vi "Linear Ramp (DBL).vi"(6 "Options":T1, 9 "Delta":dbl, 10 "Max":dbl, 11 "Min":dbl) -> (1 "# Elements":i32, 3 "Ramp":dbl[](array[numeric]))   [LabVIEW 2021, in "Arrays.lvlib"]
doc: "Creates a linear ramp with steps provided by \"Delta\".\nDepending on the chosen Options:\n\n- Include Min/Exclude Max (Default)\n- Exclude Min/Include Max\n- Include Both\n- Exclude Both\n\nthe number of array elements will vary as well as the start and end values."
uses:
  Arrays.lvlib
  Linear Ramp End Options.ctl
  Comparison/Comparison.lvlib
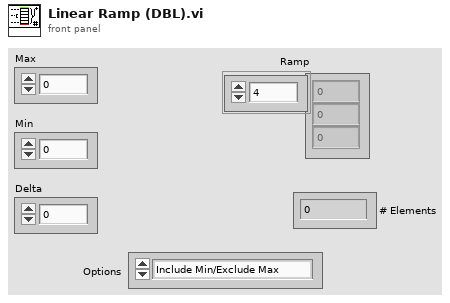
[diagram p1: front panel]
types:
  T1 = typedef "Arrays.lvlib/Linear Ramp End Options.ctl" = enum16{"Include Min/Exclude Max", "Exclude Min/Include Max", "Include Both Ends", "Exclude Both Ends"}
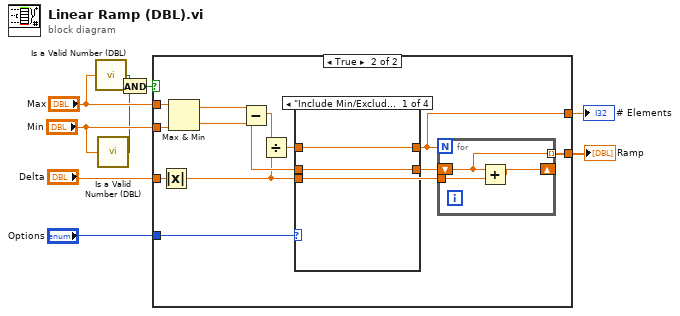
[diagram p0: block diagram]
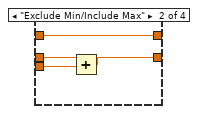
[diagram p3: hidden frame]
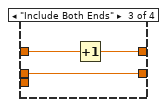
[diagram p4: hidden frame]
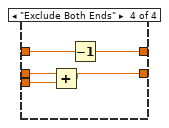
[diagram p5: hidden frame]
diagram:
  n1 = call "Is a Valid Number (DBL).vi"("Number"="Max") -> ("Valid Number?"=w2:bool)  [unwired: 8 in]
  n2 = call "Is a Valid Number (DBL).vi"("Number"="Min") -> ("Valid Number?"=w3:bool)  [unwired: 8 in]
  n3 = And(x=w2, y=w3) -> (x .and. y?=w1:bool)
  n4 = case shown="True" w1 {
    tunnel: "Delta" -> [_ w21]
    tunnel: [_ w18] -> w8
    tunnel: "Options" -> [_ w17]
    tunnel: [_ w15] -> w6
    tunnel: "Min" -> [_ w11]
    tunnel: "Max" -> [_ w10]
    frame False {
    }
    frame True {
      n5 = Absolute Value(x=w21) -> (abs(x)=w12:dbl)
      n6 = Max & Min(x=w10, y=w11) -> (max(x,y)=w19:dbl, min(x,y)=w14:dbl)
      n7 = Subtract(x=w19, y=w14) -> (x-y=w20:dbl)
      n8 = Divide(x=w20, y=w12) -> (x/y=w16:dbl)
      n9 = case shown="\"Include Min/Exclude Max\", Default" w17 {
        tunnel: w16 -> [w23 w24 w30 w35]
        tunnel: [w23 w24 w29 w34] -> w15
        tunnel: w14 -> [w22 w27 w28 w33]
        tunnel: [w22 w25 w28 w31] -> w13
        tunnel: w12 -> [_ w26 _ w32]
        frame "Include Min/Exclude Max", Default {
        }
        frame "Exclude Min/Include Max" {
          n10 = Add(x=w27, y=w26) -> (x+y=w25:dbl)
        }
        frame "Include Both Ends" {
          n11 = Increment(x=w30) -> (x+1=w29:dbl)
        }
        frame "Exclude Both Ends" {
          n12 = Add(x=w33, y=w32) -> (x+y=w31:dbl)
          n13 = Decrement(x=w35) -> (x-1=w34:dbl)
        }
      }
      n14 = for {
        N: w15 -> [_]
        shift-right: [w37] -> _
        shift-left: w13 -> [w36]
        tunnel: w12 -> [w38]
        tunnel: [w36] -> w18 mode=indexing
        n15 = Add(x=w36, y=w38) -> (x+y=w37:dbl)
      }
    }
  }
  "# Elements" <- w6
  "Ramp" <- w8
